vi "mag-field_stop_driver.vi"(0 "B-field driver ref":refnum<vi>) -> ()   [LabVIEW 2010]
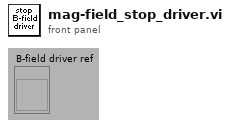
[diagram p1: front panel]
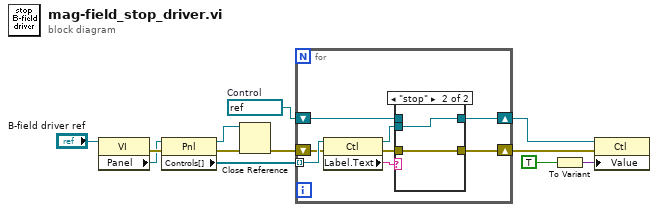
[diagram p0: block diagram]
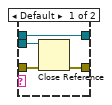
[diagram p2: hidden frame]
diagram:
  w7 = refnum<vi> refnum  # Control
  n1 = property class="VI"(reference="B-field driver ref") -> (error out=w5:errorcluster, "Panel"=w1:refnum<vi>)  [unwired: 1 in, 1 out]
  n2 = property class="Pnl"(reference=w1, error in=w5) -> (reference out=w3:refnum<vi>, error out=w4:errorcluster, "Controls[]"=w2:refnum<vi>[])
  n3 = Close Reference(reference=w3, error in (no error)=w4) -> (error out=w6:errorcluster)
  n4 = for {
    tunnel: w2 -> [w20] mode=indexing
    shift-right: [w15] -> w8
    shift-left: w6 -> [w17]
    shift-right: [w14] -> w9
    shift-left: w7 -> [w13]
    n5 = property class="Ctl"(reference=w20, error in=w17) -> (reference out=w18:refnum<vi>, error out=w16:errorcluster, "Label.Text"=w19:string)
    n6 = case shown="\"stop\"" w19 {
      tunnel: w18 -> [w21 w25]
      tunnel: w16 -> [w22 w26]
      tunnel: [w23 w26] -> w15
      tunnel: [w24 w25] -> w14
      tunnel: w13 -> [w24 _]
      frame Default {
        n7 = Close Reference(reference=w21, error in (no error)=w22) -> (error out=w23:errorcluster)
      }
      frame "stop" {
      }
    }
  }
  n8 = To Variant(anything=TRUE ("stop")) -> (Variant=w12:variant)
  n9 = property class="Ctl"(reference=w9, error in=w8, "Value"=w12) -> ()  [unwired: 2 out]
